vi "Deviation Mode.vi"() -> ()   [LabVIEW 2021]
doc: "Demonstrates how to initialize the bridge, configure measurement parameters, and perform both single and continuous measurements. Additionally this VI demonstrates configuration and execution of deviation mode measurements."
uses:
  <vilib>/Utility/file.llb/Write To Spreadsheet File (string).vi
  Andeen-Hagerling 2700A.lvlib
panel:
  in  "Clear":bool
  in  "Save":bool
  out "measurement buffer":string[](array[string])
  out "cap graph data":dbl[](array[numeric])
  out "loss graph data":dbl[](array[numeric])
  out "time graph data":timestamp[](array[timestamp])
  in  "cancel measure":bool
  in  "cancel dev init":bool
  out "Loss Analog Output":cluster{cluster{dbl, dbl}[]}[](graph)
  out "Capacitance Analog Output":cluster{cluster{dbl, dbl}[]}[](graph)
  out "aout point":T1
  in  "aout bias":T2
  in  "aout span":T3
  in  "aout source":T4 {"aout source cap" items=["DEV", "BIAS", "GROUND"]; "aout source loss" items=["DEV", "BIAS", "GROUND"]}
  in  "aout limit":T5
  in  "aout limit error":T6
  in  "aout cfactor":cluster{"cfactor cap":dbl, "cfactor loss":dbl}
  in  "aout bounds":T7
  out "Interface Information:Interface Type":u16(ring)=1 items=["GPIB"=1, "VXI"=2, "GPIB-VXI"=3, "Serial"=4, "PXI"=5, "TCPIP"=6, "USB"=7, "FireWire"=9]
  out "V 2":string
  out "Hz 2":string
  out "Capacitance Graph":cluster{timestamp[], dbl[]}(graph)
  out "Loss Graph":cluster{timestamp[], dbl[]}(graph)
  in  "Continuous":bool
  in  "dev rollofff":T8
  in  "dev format":T9
  in  "dev average":dbl
  in  "dev point auto":cluster{"cap":bool, "loss":bool}
  in  "dev fetch":bool
  in  "dev position":T10
  in  "dev bounds":T11
  out "deviation region":cluster{cluster{dbl, dbl}[]}[](graph)
  in  "dev margin":dbl
  in  "dev span":cluster{"dev span cap":dbl, "dev span loss":dbl}
  in  "dev point":T12
  out "bridge error":T13
  in  "deviation mode":bool
  out "Bridge Status":string
  out "Error Message":string
  out "V":string
  out "Hz":string
  out "pF":string
  in  "units":i32(ring)=1 items=["NS"=1, "DS"=2, "KO"=3, "GO"=4, "JP"=5]
  out "Applied Voltage":dbl format="%#_10f"
  out "Firmware Revision:":string
  in  "Maximum Applied Voltage":dbl=15.0
  in  "Average\nExponent":i32=4
  in  "Bridge Frequency":dbl=1000.0
  in  "stop":bool
  out "greater than":string
  out "Loss":dbl format="%#_10f"
  out "Measurement Frequency":dbl format="%#_10f"
  out "Capacitance":dbl format="%#_10f"
  out "measurement results":T14 {"Loss" format="%#_10f"; "Capacitance" format="%#_10f"; "Frequency" format="%#_8f"}
  in  "Measure":bool
  # "Deviation Mode Parameters"
  # "AH2700A ULTRA-PRECISION CAPACITANCE BRIDGE"
  # "Measurement Parameters"
  # "Measurement Results"
  # "Analog Out Parameters"
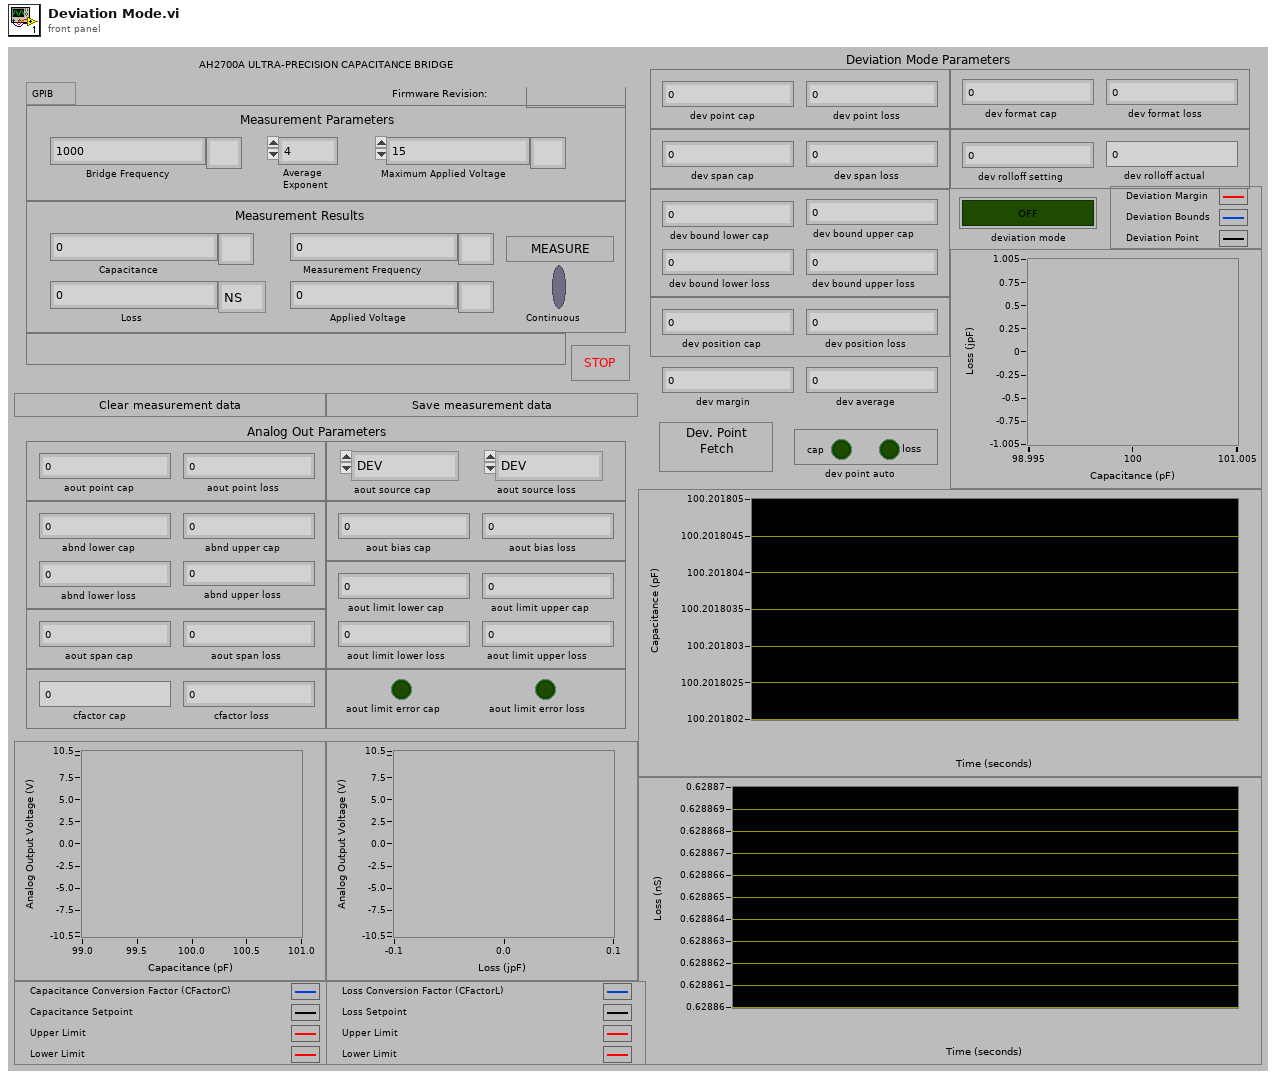
[diagram p1: front panel]
types:
  T1 = cluster{"aout point cap":dbl, "aout point loss":dbl}
  T2 = cluster{"aout bias cap":dbl, "aout bias loss":dbl}
  T3 = cluster{"aout span cap":dbl, "aout span loss":dbl}
  T4 = cluster{"aout source cap":u16, "aout source loss":u16}
  T5 = cluster{"aout limit upper cap":dbl, "aout limit upper loss":dbl, "aout limit lower cap":dbl, "aout limit lower loss":dbl}
  T6 = cluster{"aout limit error cap":bool, "aout limit error loss":bool}
  T7 = cluster{"abnd upper cap":dbl, "abnd upper loss":dbl, "abnd lower cap":dbl, "abnd lower loss":dbl}
  T8 = cluster{"dev rolloff setting":dbl, "dev rolloff actual":dbl}
  T9 = cluster{"dev format cap":i32, "dev format loss":i32}
  T10 = cluster{"dev position cap":dbl, "dev position loss":dbl}
  T11 = cluster{"dev bound upper cap":dbl, "dev bound upper loss":dbl, "dev bound lower cap":dbl, "dev bound lower loss":dbl}
  T12 = cluster{"dev point cap":dbl, "dev point loss":dbl}
  T13 = cluster{"error message":string, "error code":i32}
  T14 = cluster{"Error":i32, "Frequency":dbl, "Capacitance":dbl, "Loss":dbl, "GreaterThan":bool, "Voltage":dbl}
  T15 = cluster{"Baud Rate":u32, "Parity":u16, "Data Bits":u16, "Stop Bits":u16, "Flow Control":u16}
  T16 = cluster{"frequency":dbl, "average":i32, "voltage":dbl, "units":i32, "dev mode":bool, "dev point auto":cluster{"dev point auto cap":bool, "dev point auto loss":bool}, "dev parameters":cluster{"dev bounds":cluster{"dev bound upper cap":dbl, "dev bound upper loss":dbl, "dev bound lower cap":dbl, "dev bound lower loss":dbl}, "dev point":cluster{"dev point cap":dbl, "dev point loss":dbl}, "dev position":cluster{"dev position cap":dbl, "dev position loss":dbl}, "dev span":cluster{"dev span cap":dbl, "dev span loss":dbl}, "dev margin":dbl}, "dev average":dbl, "dev format":cluster{"dev format cap":i32, "dev format loss":i32}, "dev rollofff":cluster{"dev rolloff setting":dbl, "dev rolloff actual":dbl}, "aout bias":cluster{"ABiasC":dbl, "ABiasL":dbl}, "aout bounds":cluster{"ABndUpC":dbl, "ABndUpL":dbl, "ABndLoC":dbl, "ABndLoL":dbl}, "aout cfactor":cluster{"CFactorC":dbl, "CFactorL":dbl}, "aout limit error":cluster{"ALimErrC":bool, "ALimErrL":bool}, "aout limit":cluster{"ALimUpC":dbl, "ALimUpL":dbl, "ALimLoC":dbl, "ALimLoL":dbl}, "aout source":cluster{"ASourceC (0:DEV)":u16, "ASourceL (0:DEV)":u16}, "aout span":cluster{"ASpanC (20.0)":dbl, "ASpanL (20.0)":dbl}, "aout point":cluster{"APointC":dbl, "APointL":dbl}}
  T17 = cluster{"dev point auto cap":bool, "dev point auto loss":bool}
  T18 = cluster{"dev bounds":cluster{"dev bound upper cap":dbl, "dev bound upper loss":dbl, "dev bound lower cap":dbl, "dev bound lower loss":dbl}, "dev point":cluster{"dev point cap":dbl, "dev point loss":dbl}, "dev position":cluster{"dev position cap":dbl, "dev position loss":dbl}, "dev span":cluster{"dev span cap":dbl, "dev span loss":dbl}, "dev margin":dbl}
  T19 = cluster{"ABndUpC":dbl, "ABndUpL":dbl, "ABndLoC":dbl, "ABndLoL":dbl}
  T20 = cluster{"ALimUpC":dbl, "ALimUpL":dbl, "ALimLoC":dbl, "ALimLoL":dbl}
  T21 = cluster{"ASpanC (20.0)":dbl, "ASpanL (20.0)":dbl}
  T22 = cluster{"ASourceC (0:DEV)":u16, "ASourceL (0:DEV)":u16}
  T23 = cluster{"dev point cap":bool, "dev point loss":bool}
  T24 = cluster{"dev span cap":bool, "dev span loss":bool}
  T25 = cluster{"dev bound upper cap":bool, "dev bound upper loss":bool, "dev bound lower cap":bool, "dev bound lower loss":bool}
  T26 = cluster{"dev position cap":bool, "dev position loss":bool}
  T27 = cluster{"dev format cap":bool, "dev format loss":bool}
  T28 = cluster{"dev rolloff setting":bool, "dev rolloff actual":bool}
  T29 = cluster{"aout bias cap":bool, "aout bias loss":bool}
  T30 = cluster{"abnd upper cap":bool, "abnd upper loss":bool, "abnd lower cap":bool, "abnd lower loss":bool}
  T31 = cluster{"aout limit upper cap":bool, "aout limit upper loss":bool, "aout limit lower cap":bool, "aout limit lower loss":bool}
  T32 = cluster{"aout span cap":bool, "aout span loss":bool}
  T33 = cluster{"aout source cap":bool, "aout source loss":bool}
  T34 = cluster{"error":i32, "frequency":dbl, "capacitance":dbl, "loss":dbl, "greater than":bool, "voltage":dbl}
  T35 = cluster{"time graph data":timestamp[], "cap graph data":dbl[]}
  T36 = cluster{"time graph data":timestamp[], "loss graph data":dbl[]}
  T37 = cluster{"aout bounds":cluster{"ABndUpC":dbl, "ABndUpL":dbl, "ABndLoC":dbl, "ABndLoL":dbl}, "aout cfactor":cluster{"CFactorC":dbl, "CFactorL":dbl}, "aout span":cluster{"ASpanC":dbl, "ASpanL":dbl}, "aout point":cluster{"APointC":dbl, "APointL":dbl}}
  T38 = cluster{"error code":i32, "frequency":dbl, "capacitance":dbl, "loss":dbl, "greater than":bool, "voltage":dbl}
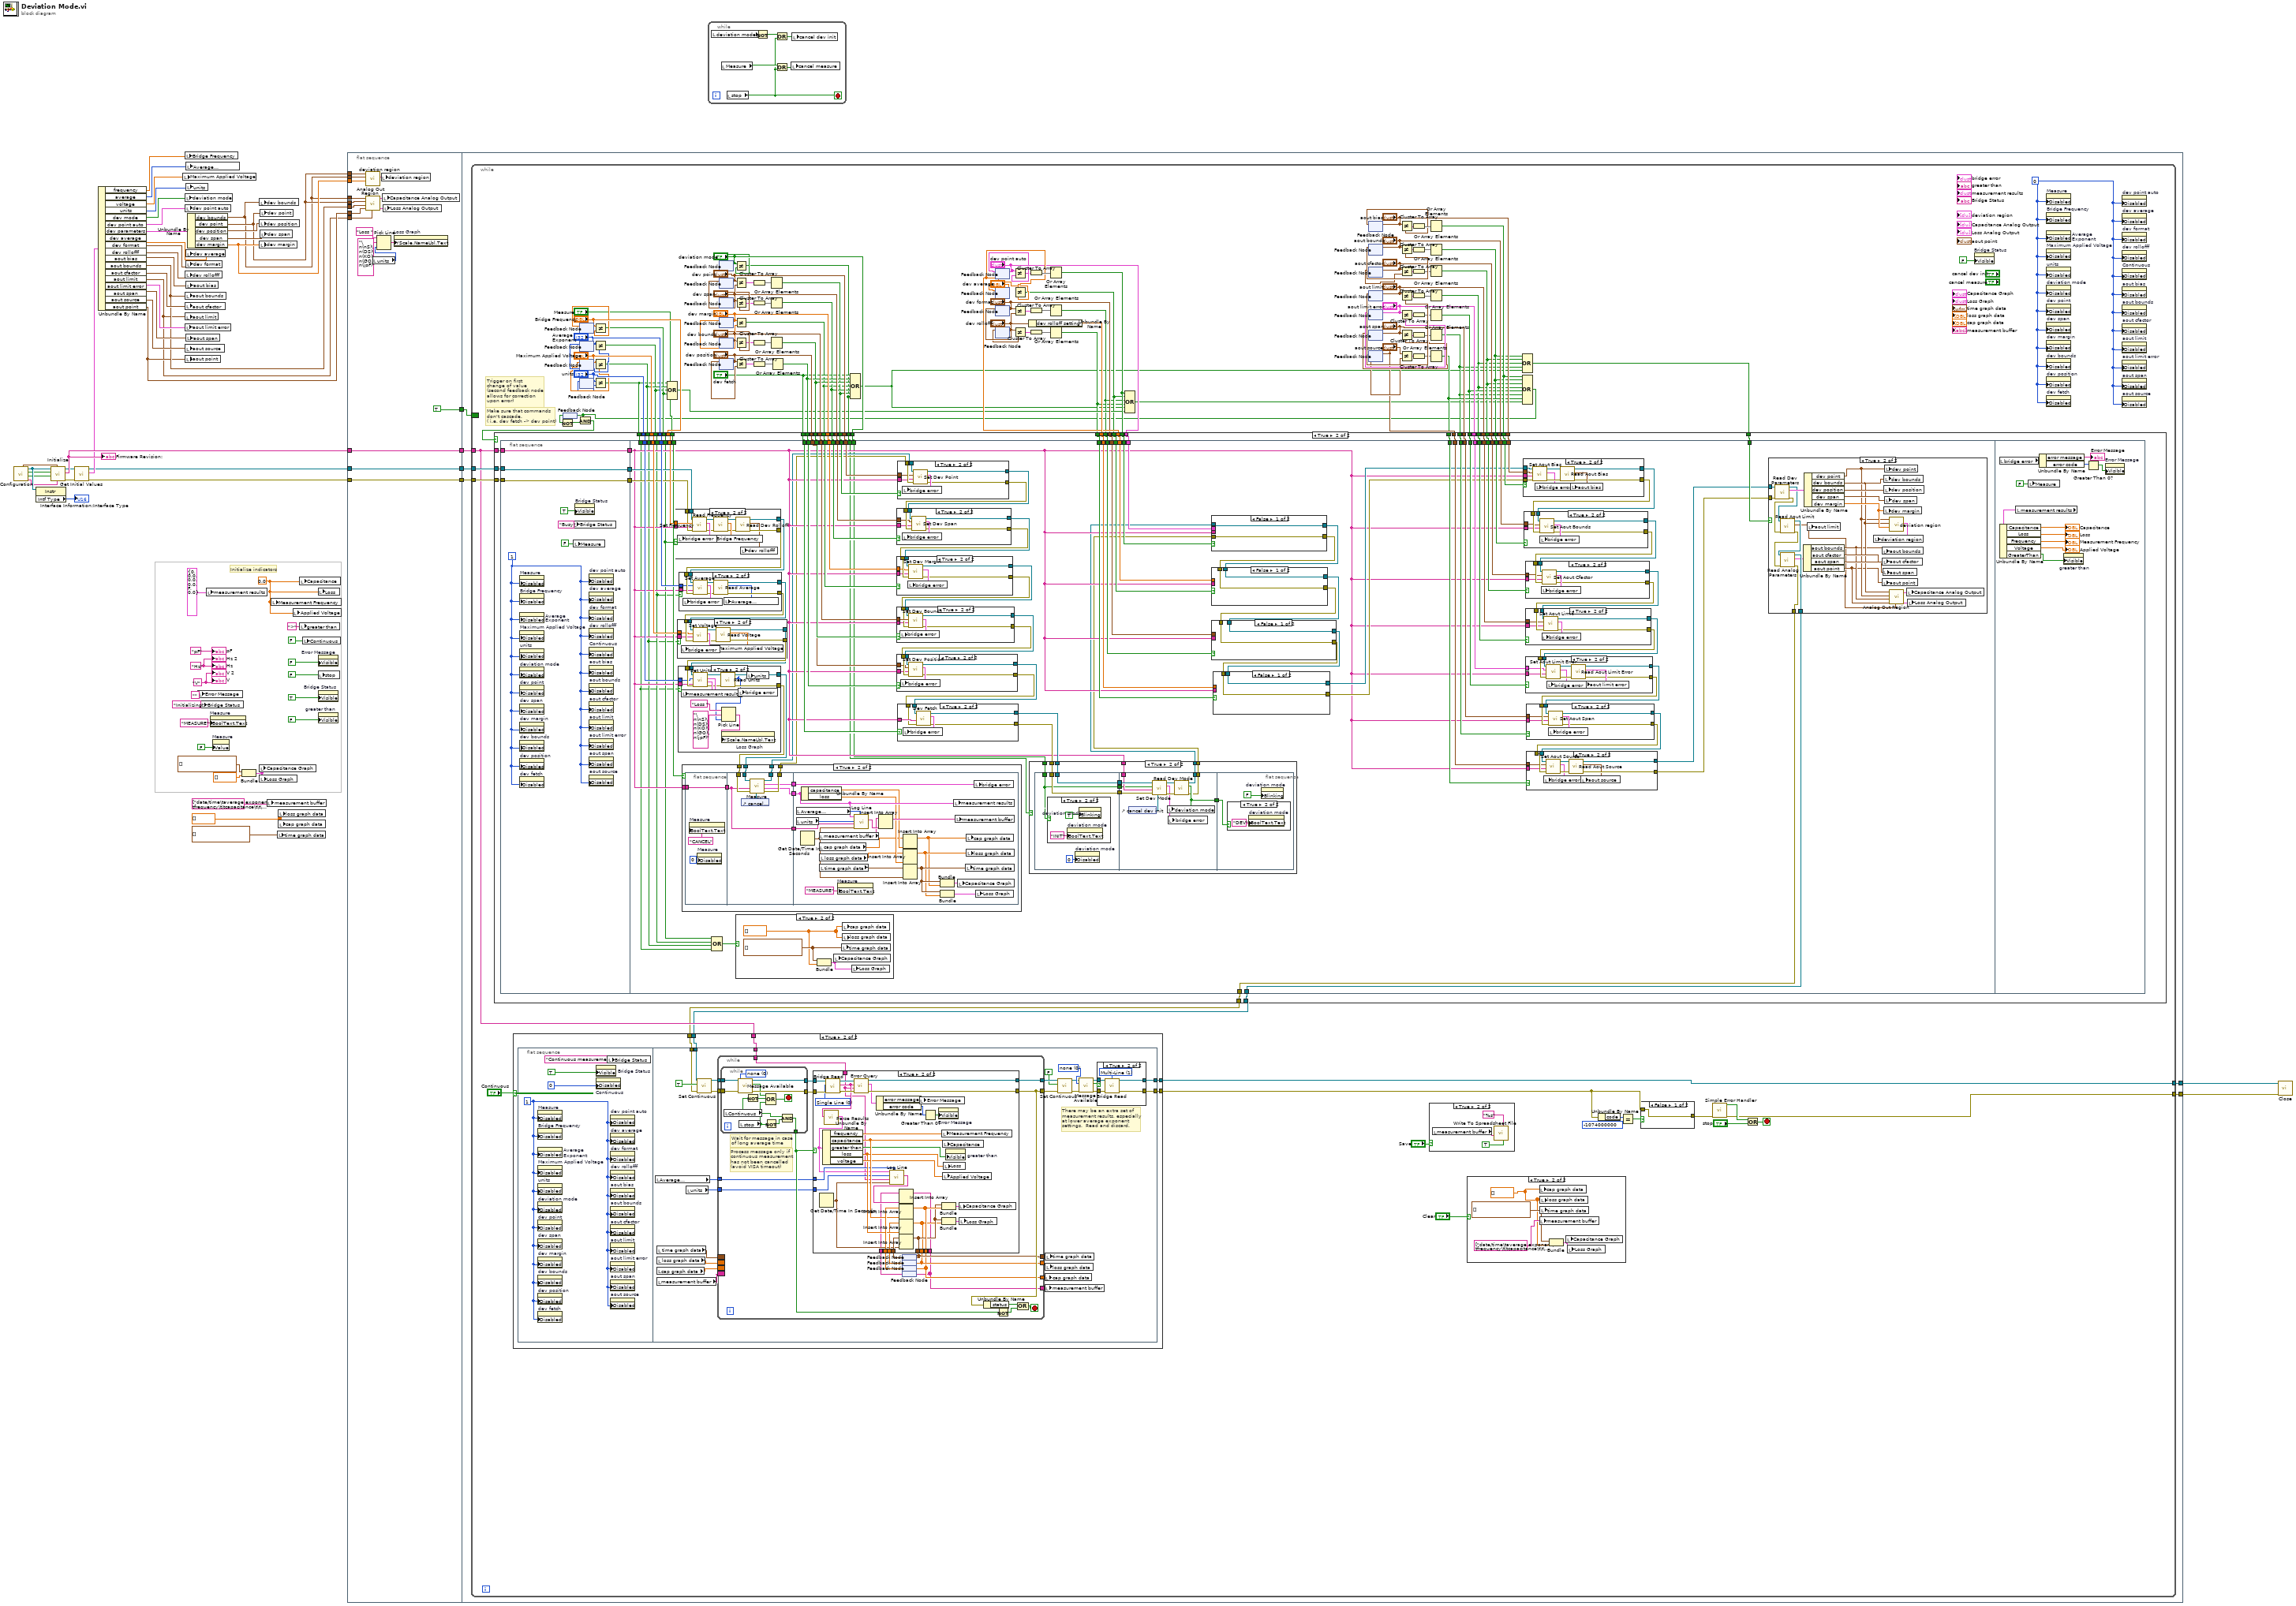
[diagram p0: block diagram]
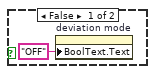
[diagram p11: hidden frame]
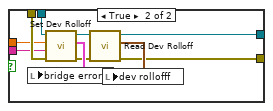
[diagram p20: hidden frame]
diagram:
  w2 = dbl[] []
  w42 = "V" ("V")
  w43 = "Hz" ("Hz")
  w57 = 0.0 ("Capacitance")
  # "Initialize indicators"
  n1 = call "Configuration.vi"() -> ("firmware version"=w9:string, "Reset"=w14:bool, "ID Query"=w10:bool, "VISA resource name out"=w41:refnum<visa-resource-name>, "serial configuration out"=w62:T15)  [unwired: 7 in]
  n2 = property class="Instr"(reference=w41) -> ("Intf Type"=→"Interface Information:Interface Type":u16)  [unwired: 1 in, 2 out]
  n3 = call "Initialize.vi"("firmware revision"=w9, "Serial Configuration"=w62, "Reset (True)"=w14, "ID Query (True)"=w10, "VISA resource name"=w41) -> ("error out"=w38:errorcluster, "firmware revision"=w47:string, "VISA resource name out"=w39:refnum<visa-resource-name>)  [unwired: 4 in]
  "Firmware Revision:" <- w47
  n4 = call "Get Initial Values.vi"("error in (no error)"=w38, "VISA resource name"=w39) -> ("error out"=w27:errorcluster, "initial values"=w37:T16, "VISA resource name out"=w26:refnum<visa-resource-name>)  [unwired: 7 in]
  n5 = Unbundle By Name(w37) -> ("frequency"=w23:dbl, "average"=w36:i32, "voltage"=w35:dbl, "units"=w34:i32, "dev mode"=w33:bool, "dev point auto"=w32:T17, "dev parameters"=w31:T18, "dev average"=w30:dbl, "dev format"=w29:T9, "dev rollofff"=w28:T8, "aout bias"=w25:cluster{"ABiasC":dbl, "ABiasL":dbl}, "aout bounds"=w18:T19, "aout cfactor"=w22:cluster{"CFactorC":dbl, "CFactorL":dbl}, "aout limit"=w16:T20, "aout limit error"=w21:cluster{"ALimErrC":bool, "ALimErrL":bool}, "aout span"=w20:T21, "aout source"=w19:T22, "aout point"=w17:cluster{"APointC":dbl, "APointL":dbl})
  n6 = local write "Maximum Applied Voltage"(w35) -> ()
  n7 = local write "Bridge Frequency"(w23) -> ()
  n8 = local write "deviation mode"(w33) -> ()
  n9 = local write "aout limit error"(w21) -> ()
  n10 = local write "dev point auto"(w32) -> ()
  n11 = local write "dev rollofff"(w28) -> ()
  n12 = local write "aout bounds"(w18) -> ()
  n13 = local write "aout cfactor"(w22) -> ()
  n14 = local write "aout limit"(w16) -> ()
  n15 = local write "aout source"(w19) -> ()
  n16 = local write "aout point"(w17) -> ()
  n17 = local write "Average\nExponent"(w36) -> ()
  n18 = local write "units"(w34) -> ()
  n19 = local write "dev average"(w30) -> ()
  n20 = local write "dev format"(w29) -> ()
  n21 = local write "aout bias"(w25) -> ()
  n22 = local write "aout span"(w20) -> ()
  n23 = Unbundle By Name(w31) -> ("dev bounds"=w6:T11, "dev point"=w7:T12, "dev position"=w49:T10, "dev span"=w48:cluster{"dev span cap":dbl, "dev span loss":dbl}, "dev margin"=w8:dbl)
  n24 = local write "Error Message"("") -> ()
  n25 = local write "Bridge Status"("Initializing" ("Error Message")) -> ()
  n26 = local write "measurement results"(T14 {"Error"=0, "Frequency"=0.0, "Capacitance"=0.0, "Loss"=0.0, "GreaterThan"=FALSE, "Voltage"=0.0} ("measurement results")) -> ()
  n27 = property on="Measure" class="Bool (strict)"("BoolText.Text"="MEASURE" ("Boolean Text.Text")) -> ()  [unwired: 2 in, 2 out]
  n28 = property on="Measure" class="Bool (strict)"("Value"=FALSE ("Measure")) -> ()  [unwired: 2 in, 2 out]
  n29 = Bundle(timestamp[] [], dbl[] []) -> (w44:cluster{timestamp[], dbl[]})  [unwired: 1 in]
  n30 = local write "Capacitance Graph"(w44) -> ()
  n31 = local write "dev bounds"(w6) -> ()
  n32 = local write "dev position"(w49) -> ()
  n33 = local write "dev margin"(w8) -> ()
  n34 = local write "Loss Graph"(w44) -> ()
  n35 = local write "dev point"(w7) -> ()
  n36 = local write "dev span"(w48) -> ()
  n37 = local write "measurement buffer"(string[] ["date/time\taverage exponent\tfrequency\t\tcapacitance\t\t\tloss\t\tvoltage\t\terror code\terror message"]) -> ()
  n38 = local write "Measurement Frequency"(w57) -> ()
  n39 = local write "time graph data"(timestamp[] []) -> ()
  n40 = local write "loss graph data"(w2) -> ()
  n41 = local write "cap graph data"(w2) -> ()
  n42 = local write "Applied Voltage"(w57) -> ()
  n43 = local write "Capacitance"(w57) -> ()
  n44 = local write "greater than"(">" ("greater than")) -> ()
  n45 = local write "Continuous"(FALSE ("Continuous")) -> ()
  n46 = local write "Loss"(w57) -> ()
  n47 = property on="Error Message" class="Str"("Visible"=FALSE) -> ()  [unwired: 2 in, 2 out]
  n48 = local write "stop"(FALSE ("stop")) -> ()
  n49 = property on="Bridge Status" class="Str"("Visible"=TRUE) -> ()  [unwired: 2 in, 2 out]
  n50 = property on="greater than" class="Str"("Visible"=FALSE) -> ()  [unwired: 2 in, 2 out]
  n51 = flat-sequence {
    tunnel: w27 -> [w79]
    tunnel: w26 -> [w80]
    tunnel: w47 -> [w81]
    tunnel: [w81] -> w52
    tunnel: [w80] -> w51
    tunnel: [w79] -> w50
    tunnel: w6 -> [w77]
    tunnel: w7 -> [w76]
    tunnel: w8 -> [w75]
    tunnel: [TRUE] -> w24
    tunnel: w6 -> [w73]
    tunnel: w7 -> [w72]
    tunnel: w18 -> [w71]
    tunnel: w17 -> [w70]
    tunnel: w16 -> [w63]
    tunnel: [w87] -> w60
    tunnel: [w86] -> w59
    tunnel: w52 -> [w85]
    tunnel: w51 -> [w84]
    tunnel: w50 -> [w83]
    tunnel: w24 -> [w82]
    frame #0 {
      n52 = call "deviation region.vi"("dev margin"=w75, "dev bounds"=w77, "dev point"=w76) -> ("deviation region"=w78:cluster{cluster{dbl, dbl}[]}[])  [unwired: 8 in]
      n53 = call "Analog Out Region.vi"("aout limit"=w63, "aout point"=w70, "aout bounds"=w71, "dev point"=w72, "dev bounds"=w73) -> ("Loss Analog Output"=w68:cluster{cluster{dbl, dbl}[]}[], "Capacitance Analog Output"=w69:cluster{cluster{dbl, dbl}[]}[])  [unwired: 5 in]
      n54 = local read "units"() -> (w65:i32)
      n55 = Pick Line(string ("")="Loss ", multi-line string="\n(nS)\n(DS)\n(KO)\n(GO)\n(jpF)", line index=w65) -> (output string=w64:string)
      n56 = local write "deviation region"(w78) -> ()
      n57 = local write "Capacitance Analog Output"(w69) -> ()
      n58 = local write "Loss Analog Output"(w68) -> ()
      n59 = property on="Loss Graph" class="XYGraph (strict)"("YScale.NameLbl.Text"=w64) -> ()  [unwired: 2 in, 2 out]
    }
    frame #1 {
      n60 = while {
        tunnel: w84 -> [w209]
        tunnel: w83 -> [w208]
        tunnel: [w204] -> w87
        tunnel: [w160] -> w86
        tunnel: w85 -> [w159]
        border: w82 -> [_]
        stop <- w205 stop-if-true
        w102 = u8 0 ("Disabled")
        # "Trigger on first\nchange of value\n(second feedback node\nallows for correction\nupon error)"
        # "Make sure that commands\ndon't cascade. \n( i.e. dev fetch -> dev point)"
        n61 = feedback #1() -> (w157:bool)
        n62 = Not(x=w157) -> (.not. x?=w158:bool)
        n63 = feedback-in #2("Bridge Frequency") -> ()
        n64 = feedback #2() -> (w192:dbl)  [unwired: 1 in]
        n65 = feedback-in #3("Average\nExponent") -> ()
        n66 = feedback #3() -> (w191:i32)  [unwired: 1 in]
        n67 = feedback-in #4("Maximum Applied Voltage") -> ()
        n68 = feedback #4() -> (w190:dbl)  [unwired: 1 in]
        n69 = feedback-in #5("units") -> ()
        n70 = feedback #5() -> (w189:i32)  [unwired: 1 in]
        n71 = Not Equal?(x="Bridge Frequency", y=w192) -> (x != y?=w150:bool)
        n72 = Not Equal?(x="Average\nExponent", y=w191) -> (x != y?=w149:bool)
        n73 = Not Equal?(x="Maximum Applied Voltage", y=w190) -> (x != y?=w151:bool)
        n74 = Not Equal?(x="units", y=w189) -> (x != y?=w148:bool)
        n75 = Compound Arithmetic op=OR(w148, w151, w149, w150, "Measure") -> (w100:bool)
        n76 = feedback-in #6("deviation mode") -> ()
        n77 = feedback #6() -> (w193:bool)  [unwired: 1 in]
        n78 = feedback-in #7("dev point") -> ()
        n79 = feedback #7() -> (w188:T12)  [unwired: 1 in]
        n80 = feedback-in #8("dev span") -> ()
        n81 = feedback #8() -> (w186:cluster{"dev span cap":dbl, "dev span loss":dbl})  [unwired: 1 in]
        n82 = feedback-in #9("dev margin") -> ()
        n83 = feedback #9() -> (w184:dbl)  [unwired: 1 in]
        n84 = feedback-in #10("dev bounds") -> ()
        n85 = feedback #10() -> (w179:T11)  [unwired: 1 in]
        n86 = feedback-in #11("dev position") -> ()
        n87 = feedback #11() -> (w176:T10)  [unwired: 1 in]
        n88 = Not Equal?(x="deviation mode", y=w193) -> (x != y?=w101:bool)
        n89 = Not Equal?(x="dev point", y=w188) -> (x != y?=w147:T23)
        n90 = Not Equal?(x="dev span", y=w186) -> (x != y?=w146:T24)
        n91 = Not Equal?(x="dev margin", y=w184) -> (x != y?=w145:bool)
        n92 = Not Equal?(x="dev bounds", y=w179) -> (x != y?=w144:T25)
        n93 = Not Equal?(x="dev position", y=w176) -> (x != y?=w143:T26)
        n94 = Cluster To Array(cluster=w147) -> (array=w187:bool[])
        n95 = Cluster To Array(cluster=w146) -> (array=w185:bool[])
        n96 = Cluster To Array(cluster=w144) -> (array=w180:bool[])
        n97 = Cluster To Array(cluster=w143) -> (array=w177:bool[])
        n98 = Or Array Elements(Boolean array=w187) -> (logical OR=w169:bool)
        n99 = Or Array Elements(Boolean array=w185) -> (logical OR=w170:bool)
        n100 = Or Array Elements(Boolean array=w180) -> (logical OR=w171:bool)
        n101 = Or Array Elements(Boolean array=w177) -> (logical OR=w172:bool)
        n102 = Compound Arithmetic op=OR("dev fetch", w172, w171, w145, w170, w169, w101) -> (w94:bool)
        n103 = feedback-in #12("dev point auto") -> ()
        n104 = feedback #12() -> (w153:cluster{"cap":bool, "loss":bool})  [unwired: 1 in]
        n105 = feedback-in #13("dev average") -> ()
        n106 = feedback #13() -> (w155:dbl)  [unwired: 1 in]
        n107 = feedback-in #14("dev format") -> ()
        n108 = feedback #14() -> (w141:T9)  [unwired: 1 in]
        n109 = feedback-in #15("dev rollofff") -> ()
        n110 = feedback #15() -> (w138:T8)  [unwired: 1 in]
        n111 = Not Equal?(x="dev point auto", y=w153) -> (x != y?=w152:cluster{"cap":bool, "loss":bool})
        n112 = Not Equal?(x="dev average", y=w155) -> (x != y?=w99:bool)
        n113 = Not Equal?(x="dev format", y=w141) -> (x != y?=w140:T27)
        n114 = Not Equal?(x="dev rollofff", y=w138) -> (x != y?=w137:T28)
        n115 = Cluster To Array(cluster=w152) -> (array=w174:bool[])
        n116 = Cluster To Array(cluster=w140) -> (array=w165:bool[])
        n117 = Unbundle By Name("dev rollofff") -> ("dev rolloff setting"=w163:dbl)
        n118 = Cluster To Array(cluster=w137) -> (array=w164:bool[])
        n119 = Or Array Elements(Boolean array=w174) -> (logical OR=w167:bool)
        n120 = Or Array Elements(Boolean array=w165) -> (logical OR=w98:bool)
        n121 = Or Array Elements(Boolean array=w164) -> (logical OR=w97:bool)
        n122 = Compound Arithmetic op=OR(w167, w99, w98, w97, w94, w100) -> (w93:bool)
        n123 = feedback-in #16("aout bias") -> ()
        n124 = feedback #16() -> (w134:T2)  [unwired: 1 in]
        n125 = feedback-in #17("aout bounds") -> ()
        n126 = feedback #17() -> (w130:T7)  [unwired: 1 in]
        n127 = feedback-in #18("aout cfactor") -> ()
        n128 = feedback #18() -> (w125:cluster{"cfactor cap":dbl, "cfactor loss":dbl})  [unwired: 1 in]
        n129 = feedback-in #19("aout limit") -> ()
        n130 = feedback #19() -> (w121:T5)  [unwired: 1 in]
        n131 = feedback-in #20("aout limit error") -> ()
        n132 = feedback #20() -> (w117:T6)  [unwired: 1 in]
        n133 = feedback-in #21("aout span") -> ()
        n134 = feedback #21() -> (w113:T3)  [unwired: 1 in]
        n135 = feedback-in #22("aout source") -> ()
        n136 = feedback #22() -> (w109:T4)  [unwired: 1 in]
        n137 = Not Equal?(x="aout bias", y=w134) -> (x != y?=w135:T29)
        n138 = Not Equal?(x="aout bounds", y=w130) -> (x != y?=w131:T30)
        n139 = Not Equal?(x="aout cfactor", y=w125) -> (x != y?=w126:cluster{"cfactor cap":bool, "cfactor loss":bool})
        n140 = Not Equal?(x="aout limit", y=w121) -> (x != y?=w122:T31)
        n141 = Not Equal?(x="aout limit error", y=w117) -> (x != y?=w118:T6)
        n142 = Not Equal?(x="aout span", y=w113) -> (x != y?=w114:T32)
        n143 = Not Equal?(x="aout source", y=w109) -> (x != y?=w110:T33)
        n144 = Cluster To Array(cluster=w135) -> (array=w136:bool[])
        n145 = Cluster To Array(cluster=w131) -> (array=w132:bool[])
        n146 = Cluster To Array(cluster=w126) -> (array=w127:bool[])
        n147 = Cluster To Array(cluster=w122) -> (array=w123:bool[])
        n148 = Cluster To Array(cluster=w118) -> (array=w119:bool[])
        n149 = Cluster To Array(cluster=w114) -> (array=w115:bool[])
        n150 = Cluster To Array(cluster=w110) -> (array=w111:bool[])
        n151 = Or Array Elements(Boolean array=w136) -> (logical OR=w128:bool)
        n152 = Or Array Elements(Boolean array=w132) -> (logical OR=w106:bool)
        n153 = Or Array Elements(Boolean array=w127) -> (logical OR=w105:bool)
        n154 = Or Array Elements(Boolean array=w123) -> (logical OR=w96:bool)
        n155 = Or Array Elements(Boolean array=w119) -> (logical OR=w104:bool)
        n156 = Or Array Elements(Boolean array=w115) -> (logical OR=w95:bool)
        n157 = Or Array Elements(Boolean array=w111) -> (logical OR=w107:bool)
        n158 = case shown="True" "Save" {
          frame False {
          }
          frame True {
            n159 = local read "measurement buffer"() -> (w214:string[])
            n160 = call-poly <vilib>:"Write To Spreadsheet File.vi"("transpose? (no:F)"=TRUE, "format (%s)"="%s", "1D data"=w214) -> ()  [unwired: 5 in, 1 out]
          }
        }
        n161 = case shown="True" "Clear" {
          frame False {
          }
          frame True {
            w210 = dbl[] []
            w213 = timestamp[] [] ("time graph data")
            n162 = local write "cap graph data"(w210) -> ()
            n163 = local write "measurement buffer"(string[] ["date/time\taverage exponent\tfrequency\t\tcapacitance\t\t\tloss\t\tvoltage\t\terror code\terror message"]) -> ()
            n164 = local write "loss graph data"(w210) -> ()
            n165 = local write "time graph data"(w213) -> ()
            n166 = Bundle("time graph data"=w213, w210) -> (w212:cluster{"time graph data":timestamp[], dbl[]})  [unwired: 1 in]
            n167 = local write "Capacitance Graph"(w212) -> ()
            n168 = local write "Loss Graph"(w212) -> ()
          }
        }
        n169 = Compound Arithmetic op=OR(w106, w105, w96, w95, w94) -> (w103:bool)
        n170 = Compound Arithmetic op=OR(w128, w106, w105, w96, w104, w95, w107, w93) -> (w92:bool)
        n171 = feedback-in #1(w92) -> ()
        n172 = And(x=w92, y=w158) -> (x .and. y?=w166:bool)
        n173 = case shown="True" w166 {
          tunnel: w209 -> [w334 w386]
          tunnel: w208 -> [w335 w385]
          tunnel: "Measure" -> [_ w384]
          tunnel: w150 -> [_ w383]
          tunnel: "Bridge Frequency" -> [_ w382]
          tunnel: "Average\nExponent" -> [_ w381]
          tunnel: w149 -> [_ w380]
          tunnel: "Maximum Applied Voltage" -> [_ w379]
          tunnel: w151 -> [_ w378]
          tunnel: "units" -> [_ w377]
          tunnel: w148 -> [_ w376]
          tunnel: w159 -> [_ w374]
          tunnel: w101 -> [_ w373]
          tunnel: "deviation mode" -> [_ w372]
          tunnel: "dev point" -> [_ w371]
          tunnel: w169 -> [_ w370]
          tunnel: "dev span" -> [_ w369]
          tunnel: w170 -> [_ w368]
          tunnel: "dev margin" -> [_ w367]
          tunnel: w145 -> [_ w366]
          tunnel: "dev bounds" -> [_ w365]
          tunnel: w171 -> [_ w364]
          tunnel: "dev position" -> [_ w363]
          tunnel: w172 -> [_ w362]
          tunnel: "dev point auto" -> [_ w361]
          tunnel: w167 -> [_ w360]
          tunnel: "dev fetch" -> [_ w359]
          tunnel: "dev average" -> [_ w358]
          tunnel: w99 -> [_ w357]
          tunnel: "dev format" -> [_ w356]
          tunnel: w98 -> [_ w355]
          tunnel: w163 -> [_ w354]
          tunnel: w97 -> [_ w353]
          tunnel: [w334 w352] -> w89
          tunnel: [w335 w351] -> w88
          tunnel: "aout bias" -> [_ w350]
          tunnel: w128 -> [_ w349]
          tunnel: "aout bounds" -> [_ w348]
          tunnel: w106 -> [_ w347]
          tunnel: "aout cfactor" -> [_ w346]
          tunnel: w105 -> [_ w345]
          tunnel: "aout limit" -> [_ w344]
          tunnel: w96 -> [_ w343]
          tunnel: "aout limit error" -> [_ w342]
          tunnel: w104 -> [_ w341]
          tunnel: "aout span" -> [_ w340]
          tunnel: w95 -> [_ w339]
          tunnel: "aout source" -> [_ w338]
          tunnel: w107 -> [_ w337]
          tunnel: w103 -> [_ w336]
          frame False {
          }
          frame True {
            n174 = flat-sequence {
              tunnel: w385 -> [w394]
              tunnel: w386 -> [w395]
              tunnel: [w395] -> w388
              tunnel: [w394] -> w387
              tunnel: [w392] -> w375
              tunnel: w374 -> [w392]
              tunnel: w384 -> [w410]
              tunnel: w388 -> [w414]
              tunnel: w387 -> [w413]
              tunnel: w383 -> [w399]
              tunnel: w382 -> [w492]
              tunnel: w381 -> [w491]
              tunnel: w380 -> [w398]
              tunnel: w379 -> [w488]
              tunnel: w378 -> [w397]
              tunnel: w377 -> [w484]
              tunnel: w376 -> [w396]
              tunnel: w375 -> [w407]
              tunnel: w373 -> [w403]
              tunnel: w372 -> [w404]
              tunnel: w371 -> [w482]
              tunnel: w370 -> [w481]
              tunnel: w369 -> [w478]
              tunnel: w368 -> [w477]
              tunnel: w367 -> [w474]
              tunnel: w366 -> [w473]
              tunnel: w365 -> [w472]
              tunnel: w364 -> [w469]
              tunnel: w363 -> [w468]
              tunnel: w362 -> [w467]
              tunnel: w361 -> [w464]
              tunnel: w360 -> [w463]
              tunnel: w359 -> [w460]
              tunnel: w358 -> [w459]
              tunnel: w357 -> [w456]
              tunnel: w356 -> [w453]
              tunnel: w355 -> [w452]
              tunnel: w354 -> [w451]
              tunnel: w353 -> [w450]
              tunnel: [w415] -> w352
              tunnel: [w416] -> w351
              tunnel: w350 -> [w447]
              tunnel: w349 -> [w446]
              tunnel: w348 -> [w443]
              tunnel: w347 -> [w442]
              tunnel: w346 -> [w439]
              tunnel: w345 -> [w438]
              tunnel: w344 -> [w435]
              tunnel: w343 -> [w434]
              tunnel: w342 -> [w431]
              tunnel: w341 -> [w430]
              tunnel: w340 -> [w427]
              tunnel: w339 -> [w426]
              tunnel: w338 -> [w423]
              tunnel: w337 -> [w422]
              tunnel: w336 -> [w419]
              frame #0 {
                w390 = u8 1 ("Disabled")
                n175 = property on="Measure" class="Bool (strict)"("Disabled"=w390) -> ()  [unwired: 2 in, 2 out]
                n176 = property on="Bridge Frequency" class="DigNum (strict)"("Disabled"=w390) -> ()  [unwired: 2 in, 2 out]
                n177 = property on="Average\nExponent" class="DigNum (strict)"("Disabled"=w390) -> ()  [unwired: 2 in, 2 out]
                n178 = property on="Maximum Applied Voltage" class="DigNum (strict)"("Disabled"=w390) -> ()  [unwired: 2 in, 2 out]
                n179 = property on="units" class="Ring (strict)"("Disabled"=w390) -> ()  [unwired: 2 in, 2 out]
                n180 = property on="deviation mode" class="Bool (strict)"("Disabled"=w390) -> ()  [unwired: 2 in, 2 out]
                n181 = property on="dev point" class="Clust (strict)"("Disabled"=w390) -> ()  [unwired: 2 in, 2 out]
                n182 = property on="dev span" class="Clust (strict)"("Disabled"=w390) -> ()  [unwired: 2 in, 2 out]
                n183 = property on="dev margin" class="DigNum (strict)"("Disabled"=w390) -> ()  [unwired: 2 in, 2 out]
                n184 = property on="dev bounds" class="Clust (strict)"("Disabled"=w390) -> ()  [unwired: 2 in, 2 out]
                n185 = property on="dev position" class="Clust (strict)"("Disabled"=w390) -> ()  [unwired: 2 in, 2 out]
                n186 = property on="dev fetch" class="Bool"("Disabled"=w390) -> ()  [unwired: 2 in, 2 out]
                n187 = local write "Bridge Status"("Busy" ("Bridge Status")) -> ()
                n188 = local write "Measure"(FALSE ("Measure")) -> ()
                n189 = property on="Bridge Status" class="Str"("Visible"=TRUE) -> ()  [unwired: 2 in, 2 out]
                n190 = property on="dev point auto" class="Clust (strict)"("Disabled"=w390) -> ()  [unwired: 2 in, 2 out]
                n191 = property on="dev average" class="DigNum (strict)"("Disabled"=w390) -> ()  [unwired: 2 in, 2 out]
                n192 = property on="dev format" class="Clust (strict)"("Disabled"=w390) -> ()  [unwired: 2 in, 2 out]
                n193 = property on="dev rollofff" class="Clust (strict)"("Disabled"=w390) -> ()  [unwired: 2 in, 2 out]
                n194 = property on="Continuous" class="Bool (strict)"("Disabled"=w390) -> ()  [unwired: 2 in, 2 out]
                n195 = property on="aout bias" class="Clust (strict)"("Disabled"=w390) -> ()  [unwired: 2 in, 2 out]
                n196 = property on="aout bounds" class="Clust (strict)"("Disabled"=w390) -> ()  [unwired: 2 in, 2 out]
                n197 = property on="aout cfactor" class="Clust (strict)"("Disabled"=w390) -> ()  [unwired: 2 in, 2 out]
                n198 = property on="aout limit" class="Clust (strict)"("Disabled"=w390) -> ()  [unwired: 2 in, 2 out]
                n199 = property on="aout limit error" class="Clust (strict)"("Disabled"=w390) -> ()  [unwired: 2 in, 2 out]
                n200 = property on="aout span" class="Clust (strict)"("Disabled"=w390) -> ()  [unwired: 2 in, 2 out]
                n201 = property on="aout source" class="Clust (strict)"("Disabled"=w390) -> ()  [unwired: 2 in, 2 out]
              }
              frame #1 {
                n202 = case shown="True" w399 {
                  tunnel: w492 -> [_ w781]
                  tunnel: w414 -> [w768 w780]
                  tunnel: w413 -> [w767 w779]
                  tunnel: w407 -> [_ w778]
                  tunnel: [w768 w771] -> w490
                  tunnel: [w767 w770] -> w489
                  frame False {
                  }
                  frame True {
                    n203 = call "Set Frequency.vi"("error in (no error)"=w779, "firmware revision"=w778, "frequency (1000)"=w781, "VISA resource name"=w780) -> ("error out"=w775:errorcluster, "bridge error"=w777:T13, "VISA resource name out"=w776:refnum<visa-resource-name>)  [unwired: 5 in]
                    n204 = local write "bridge error"(w777) -> ()
                    n205 = call "Read Frequency.vi"("error in (no error)"=w775, "VISA resource name"=w776) -> ("error out"=w772:errorcluster, "frequency"=w774:dbl, "VISA resource name out"=w773:refnum<visa-resource-name>)  [unwired: 7 in]
                    n206 = local write "Bridge Frequency"(w774) -> ()
                    n207 = call "Read Dev Rolloff.vi"("error in (no error)"=w772, "VISA resource name"=w773) -> ("error out"=w770:errorcluster, "dev rollofff"=w769:T8, "VISA resource name out"=w771:refnum<visa-resource-name>)  [unwired: 7 in]
                    n208 = local write "dev rollofff"(w769) -> ()
                  }
                }
                n209 = case shown="True" w398 {
                  tunnel: w490 -> [w756 w766]
                  tunnel: w489 -> [w755 w765]
                  tunnel: [w756 w758] -> w486
                  tunnel: [w755 w760] -> w487
                  tunnel: w491 -> [_ w764]
                  tunnel: w407 -> [_ w763]
                  frame False {
                  }
                  frame True {
                    n210 = call "Set Average.vi"("error in (no error)"=w765, "firmware revision"=w763, "average (4)"=w764, "VISA resource name"=w766) -> ("error out"=w761:errorcluster, "bridge error"=w762:T13, "VISA resource name out"=w759:refnum<visa-resource-name>)  [unwired: 5 in]
                    n211 = local write "bridge error"(w762) -> ()
                    n212 = call "Read Average.vi"("error in (no error)"=w761, "VISA resource name"=w759) -> ("error out"=w760:errorcluster, "average"=w757:i32, "VISA resource name out"=w758:refnum<visa-resource-name>)  [unwired: 7 in]
                    n213 = local write "Average\nExponent"(w757) -> ()
                  }
                }
                n214 = case shown="True" w397 {
                  tunnel: w486 -> [w744 w754]
                  tunnel: w487 -> [w743 w753]
                  tunnel: [w744 w748] -> w483
                  tunnel: [w743 w746] -> w485
                  tunnel: w407 -> [_ w752]
                  tunnel: w488 -> [_ w751]
                  frame False {
                  }
                  frame True {
                    n215 = call "Set Voltage.vi"("error in (no error)"=w753, "firmware revision"=w752, "voltage (15)"=w751, "VISA resource name"=w754) -> ("error out"=w747:errorcluster, "bridge error"=w750:T13, "VISA resource name out"=w749:refnum<visa-resource-name>)  [unwired: 5 in]
                    n216 = local write "bridge error"(w750) -> ()
                    n217 = call "Read Voltage.vi"("error in (no error)"=w747, "VISA resource name"=w749) -> ("error out"=w746:errorcluster, "voltage"=w745:dbl, "VISA resource name out"=w748:refnum<visa-resource-name>)  [unwired: 7 in]
                    n218 = local write "Maximum Applied Voltage"(w745) -> ()
                  }
                }
                n219 = case shown="True" w396 {
                  tunnel: w483 -> [w728 w742]
                  tunnel: w485 -> [w727 w741]
                  tunnel: [w728 w733] -> w411
                  tunnel: [w727 w735] -> w412
                  tunnel: w407 -> [_ w740]
                  tunnel: w484 -> [_ w739]
                  frame False {
                  }
                  frame True {
                    n220 = call "Set Units.vi"("error in (no error)"=w741, "firmware revision"=w740, "units (NS)"=w739, "VISA resource name"=w742) -> ("error out"=w736:errorcluster, "measurement results"=w738:T14, "bridge error"=w737:T13, "VISA resource name out"=w734:refnum<visa-resource-name>)  [unwired: 4 in]
                    n221 = local write "measurement results"(w738) -> ()
                    n222 = call "Read Units.vi"("error in (no error)"=w736, "VISA resource name"=w734) -> ("error out"=w735:errorcluster, "units"=w730:i32, "VISA resource name out"=w733:refnum<visa-resource-name>)  [unwired: 7 in]
                    n223 = Pick Line(string ("")="Loss ", multi-line string="\n(nS)\n(DS)\n(KO)\n(GO)\n(jpF)", line index=w730) -> (output string=w729:string)
                    n224 = property on="Loss Graph" class="XYGraph (strict)"("YScale.NameLbl.Text"=w729) -> ()  [unwired: 2 in, 2 out]
                    n225 = local write "bridge error"(w737) -> ()
                    n226 = local write "units"(w730) -> ()
                  }
                }
                n227 = case shown="True" w410 {
                  tunnel: w407 -> [_ w792]
                  tunnel: w412 -> [w783 w790]
                  tunnel: w411 -> [w782 w789]
                  tunnel: [w782 w788] -> w405
                  tunnel: [w783 w787] -> w406
                  frame False {
                  }
                  frame True {
                    n228 = flat-sequence {
                      tunnel: w792 -> [w793]
                      tunnel: [w793] -> w791
                      tunnel: w791 -> [w796]
                      tunnel: w790 -> [w803]
                      tunnel: w789 -> [w802]
                      tunnel: [w801] -> w788
                      tunnel: [w800] -> w787
                      tunnel: [w798] -> w786
                      tunnel: [w797] -> w785
                      tunnel: [w796] -> w784
                      tunnel: w786 -> [w819]
                      tunnel: w785 -> [w822]
                      tunnel: w784 -> [w818]
                      frame #0 {
                        n229 = property on="Measure" class="Bool (strict)"("BoolText.Text"="CANCEL" ("Label.Text")) -> ()  [unwired: 2 in, 2 out]
                        n230 = property on="Measure" class="Bool (strict)"("Disabled"=u8 0) -> ()  [unwired: 2 in, 2 out]
                      }
                      frame #1 {
                        n231 = control-ref of="cancel measure"() -> (w799:refnum<vi>)
                        n232 = call "Measure.vi"("cancel refnum"=w799, "error in (no error)"=w803, "firmware revision"=w796, "VISA resource name"=w802) -> ("error out"=w800:errorcluster, "measurement results"=w798:T34, "bridge error"=w797:T13, "VISA resource name out"=w801:refnum<visa-resource-name>)  [unwired: 3 in]
                      }
                      frame #2 {
                        n233 = local read "Average\nExponent"() -> (w821:i32)
                        n234 = local read "units"() -> (w820:i32)
                        n235 = Get Date/Time In Seconds() -> (seconds since 1Jan1904=w812:timestamp)
                        n236 = Unbundle By Name(w819) -> ("capacitance"=w814:dbl, "loss"=w813:dbl)
                        n237 = local read "measurement buffer"() -> (w816:string[])
                        n238 = local read "cap graph data"() -> (w811:dbl[])
                        n239 = local read "loss graph data"() -> (w810:dbl[])
                        n240 = local read "time graph data"() -> (w809:timestamp[])
                        n241 = property on="Measure" class="Bool (strict)"("BoolText.Text"="MEASURE" ("Label.Text")) -> ()  [unwired: 2 in, 2 out]
                        n242 = call "Log Line.vi"("average exponent"=w821, "current time"=w812, "firmware revision"=w818, "units"=w820, "measurement results"=w819) -> ("log line"=w817:string)  [unwired: 6 in]
                        n243 = Insert Into Array(array=w816, new element=w817) -> (w815:string[])  [unwired: 1 in]
                        n244 = Insert Into Array(array=w811, new element=w814) -> (w806:dbl[])  [unwired: 1 in]
                        n245 = Insert Into Array(array=w810, new element=w813) -> (w807:dbl[])  [unwired: 1 in]
                        n246 = Insert Into Array(array=w809, new element=w812) -> (w808:timestamp[])  [unwired: 1 in]
                        n247 = Bundle("time graph data"=w808, "cap graph data"=w806) -> (w805:T35)  [unwired: 1 in]
                        n248 = Bundle("time graph data"=w808, "loss graph data"=w807) -> (w804:T36)  [unwired: 1 in]
                        n249 = local write "measurement results"(w819) -> ()
                        n250 = local write "measurement buffer"(w815) -> ()
                        n251 = local write "Capacitance Graph"(w805) -> ()
                        n252 = local write "time graph data"(w808) -> ()
                        n253 = local write "cap graph data"(w806) -> ()
                        n254 = local write "loss graph data"(w807) -> ()
                        n255 = local write "bridge error"(w822) -> ()
                        n256 = local write "Loss Graph"(w804) -> ()
                      }
                    }
                  }
                }
                n257 = Compound Arithmetic op=OR(w399, w398, w397, w396) -> (w400:bool)
                n258 = case shown="True" w400 {
                  frame False {
                  }
                  frame True {
                    w493 = dbl[] []
                    w494 = timestamp[] [] ("time graph data")
                    n259 = Bundle("time graph data"=w494, w493) -> (w495:cluster{"time graph data":timestamp[], dbl[]})  [unwired: 1 in]
                    n260 = local write "Capacitance Graph"(w495) -> ()
                    n261 = local write "time graph data"(w494) -> ()
                    n262 = local write "cap graph data"(w493) -> ()
                    n263 = local write "loss graph data"(w493) -> ()
                    n264 = local write "Loss Graph"(w495) -> ()
                  }
                }
                n265 = case shown="True" w481 {
                  tunnel: w405 -> [w718 w725]
                  tunnel: w406 -> [w719 w724]
                  tunnel: [w718 w721] -> w480
                  tunnel: [w719 w720] -> w479
                  tunnel: w482 -> [_ w723]
                  tunnel: w407 -> [_ w722]
                  frame False {
                  }
                  frame True {
                    n266 = call "Set Dev Point.vi"("error in (no error)"=w724, "firmware revision"=w722, "dev point"=w723, "VISA resource name"=w725) -> ("error out"=w720:errorcluster, "bridge error"=w726:T13, "VISA resource name out"=w721:refnum<visa-resource-name>)  [unwired: 5 in]
                    n267 = local write "bridge error"(w726) -> ()
                  }
                }
                n268 = case shown="True" w477 {
                  tunnel: w480 -> [w710 w716]
                  tunnel: w479 -> [w709 w715]
                  tunnel: [w710 w711] -> w476
                  tunnel: [w709 w712] -> w475
                  tunnel: w407 -> [_ w714]
                  tunnel: w478 -> [_ w713]
                  frame False {
                  }
                  frame True {
                    n269 = call "Set Dev Span.vi"("error in (no error)"=w715, "firmware revision"=w714, "dev span"=w713, "VISA resource name"=w716) -> ("error out"=w712:errorcluster, "bridge error"=w717:T13, "VISA resource name out"=w711:refnum<visa-resource-name>)  [unwired: 5 in]
                    n270 = local write "bridge error"(w717) -> ()
                  }
                }
                n271 = case shown="True" w473 {
                  tunnel: w476 -> [w701 w707]
                  tunnel: [w701 w702] -> w470
                  tunnel: [w700 w703] -> w471
                  tunnel: w475 -> [w700 w706]
                  tunnel: w407 -> [_ w705]
                  tunnel: w474 -> [_ w704]
                  frame False {
                  }
                  frame True {
                    n272 = call "Set Dev Margin.vi"("error in (no error)"=w706, "firmware revision"=w705, "dev margin (1.0)"=w704, "VISA resource name"=w707) -> ("error out"=w703:errorcluster, "bridge error"=w708:T13, "VISA resource name out"=w702:refnum<visa-resource-name>)  [unwired: 5 in]
                    n273 = local write "bridge error"(w708) -> ()
                  }
                }
                n274 = case shown="True" w469 {
                  tunnel: w472 -> [_ w699]
                  tunnel: w470 -> [w692 w698]
                  tunnel: w471 -> [w691 w697]
                  tunnel: w407 -> [_ w696]
                  tunnel: [w691 w694] -> w466
                  tunnel: [w692 w693] -> w465
                  frame False {
                  }
                  frame True {
                    n275 = call "Set Dev Bounds.vi"("error in (no error)"=w697, "firmware revision"=w696, "dev bounds"=w699, "VISA resource name"=w698) -> ("error out"=w694:errorcluster, "bridge error"=w695:T13, "VISA resource name out"=w693:refnum<visa-resource-name>)  [unwired: 4 in]
                    n276 = local write "bridge error"(w695) -> ()
                  }
                }
                n277 = case shown="True" w467 {
                  tunnel: w465 -> [w683 w690]
                  tunnel: w466 -> [w682 w689]
                  tunnel: w407 -> [_ w687]
                  tunnel: w468 -> [_ w686]
                  tunnel: [w682 w684] -> w461
                  tunnel: [w683 w685] -> w462
                  frame False {
                  }
                  frame True {
                    n278 = call "Set Dev Position.vi"("error in (no error)"=w689, "firmware revision"=w687, "dev position"=w686, "VISA resource name"=w690) -> ("error out"=w684:errorcluster, "bridge error"=w688:T13, "VISA resource name out"=w685:refnum<visa-resource-name>)  [unwired: 5 in]
                    n279 = local write "bridge error"(w688) -> ()
                  }
                }
                n280 = case shown="True" w460 {
                  tunnel: w407 -> [_ w681]
                  tunnel: [w675 w677] -> w408
                  tunnel: [w674 w676] -> w409
                  tunnel: w462 -> [w675 w679]
                  tunnel: w461 -> [w674 w678]
                  frame False {
                  }
                  frame True {
                    n281 = call "Dev Fetch.vi"("error in (no error)"=w678, "firmware revision"=w681, "VISA resource name"=w679) -> ("error out"=w676:errorcluster, "bridge error"=w680:T13, "VISA resource name out"=w677:refnum<visa-resource-name>)  [unwired: 6 in]
                    n282 = local write "bridge error"(w680) -> ()
                  }
                }
                n283 = case shown="True" w403 {
                  tunnel: w409 -> [w496 w507]
                  tunnel: w408 -> [w497 w505]
                  tunnel: w407 -> [_ w503]
                  tunnel: w404 -> [_ w502]
                  tunnel: [w497 w499] -> w402
                  tunnel: [w496 w498] -> w401
                  frame False {
                  }
                  frame True {
                    n284 = flat-sequence {
                      tunnel: w507 -> [w510]
                      tunnel: [w510] -> w506
                      tunnel: w505 -> [w511]
                      tunnel: [w511] -> w504
                      tunnel: w502 -> [w509]
                      tunnel: [w509] -> w500
                      tunnel: w506 -> [w521]
                      tunnel: w504 -> [w520]
                      tunnel: w503 -> [w519]
                      tunnel: [w518] -> w501
                      tunnel: w500 -> [w517]
                      tunnel: [w515] -> w499
                      tunnel: [w514] -> w498
                      tunnel: w501 -> [w525]
                      frame #0 {
                        n285 = case shown="True" w509 {
                          frame False {
                          }
                          frame True {
                            n286 = property on="deviation mode" class="Bool (strict)"("BoolText.Text"="INIT" ("Boolean Text.Text")) -> ()  [unwired: 2 in, 2 out]
                            n287 = property on="deviation mode" class="Bool (strict)"("Blinking"=TRUE) -> ()  [unwired: 2 in, 2 out]
                          }
                        }
                        n288 = property on="deviation mode" class="Bool (strict)"("Disabled"=u8 0) -> ()  [unwired: 2 in, 2 out]
                      }
                      frame #1 {
                        n289 = control-ref of="cancel dev init"() -> (w516:refnum<vi>)
                        n290 = call "Set Dev Mode.vi"("cancel refnum"=w516, "error in (no error)"=w521, "firmware revision"=w519, "dev mode"=w517, "VISA resource name"=w520) -> ("error out"=w524:errorcluster, "bridge error"=w522:T13, "VISA resource name out"=w523:refnum<visa-resource-name>)  [unwired: 4 in]
                        n291 = local write "bridge error"(w522) -> ()
                        n292 = call "Read Dev Mode.vi"("error in (no error)"=w524, "VISA resource name"=w523) -> ("error out"=w514:errorcluster, "dev mode"=w518:bool, "VISA resource name out"=w515:refnum<visa-resource-name>)  [unwired: 7 in]
                        n293 = local write "deviation mode"(w518) -> ()
                      }
                      frame #2 {
                        n294 = case shown="True" w525 {
                          frame False {
                            n295 = property on="deviation mode" class="Bool (strict)"("BoolText.Text"="OFF" ("Boolean Text.Text")) -> ()  [unwired: 2 in, 2 out]
                          }
                          frame True {
                            n296 = property on="deviation mode" class="Bool (strict)"("BoolText.Text"="DEV" ("Boolean Text.Text")) -> ()  [unwired: 2 in, 2 out]
                          }
                        }
                        n297 = property on="deviation mode" class="Bool (strict)"("Blinking"=FALSE) -> ()  [unwired: 2 in, 2 out]
                      }
                    }
                  }
                }
                n298 = case shown="False" w463 {
                  tunnel: w407 -> [_ w673]
                  tunnel: w464 -> [_ w669]
                  tunnel: [w662 w667] -> w458
                  tunnel: [w663 w666] -> w457
                  tunnel: w402 -> [w663 w665]
                  tunnel: w401 -> [w662 w664]
                  frame False {
                  }
                  frame True {
                    n299 = call "Set Dev Auto.vi"("error in (no error)"=w664, "firmware revision"=w673, "dev point auto (F/F)"=w669, "VISA resource name"=w665) -> ("error out"=w672:errorcluster, "bridge error"=w670:T13, "VISA resource name out"=w671:refnum<visa-resource-name>)  [unwired: 5 in]
                    n300 = local write "bridge error"(w670) -> ()
                    n301 = call "Read Dev Auto.vi"("error in (no error)"=w672, "VISA resource name"=w671) -> ("error out"=w667:errorcluster, "dev point auto"=w668:T17, "VISA resource name out"=w666:refnum<visa-resource-name>)  [unwired: 7 in]
                    n302 = local write "dev point auto"(w668) -> ()
                  }
                }
                n303 = case shown="False" w456 {
                  tunnel: w457 -> [w651 w661]
                  tunnel: w458 -> [w650 w660]
                  tunnel: w407 -> [_ w659]
                  tunnel: w459 -> [_ w658]
                  tunnel: [w650 w653] -> w454
                  tunnel: [w651 w652] -> w455
                  frame False {
                  }
                  frame True {
                    n304 = call "Set Dev Average.vi"("error in (no error)"=w660, "firmware revision"=w659, "dev average (0)"=w658, "VISA resource name"=w661) -> ("error out"=w657:errorcluster, "bridge error"=w655:T13, "VISA resource name out"=w656:refnum<visa-resource-name>)  [unwired: 5 in]
                    n305 = local write "bridge error"(w655) -> ()
                    n306 = call "Read Dev Average.vi"("error in (no error)"=w657, "VISA resource name"=w656) -> ("error out"=w653:errorcluster, "dev average"=w654:dbl, "VISA resource name out"=w652:refnum<visa-resource-name>)  [unwired: 7 in]
                    n307 = local write "dev average"(w654) -> ()
                  }
                }
                n308 = case shown="False" w452 {
                  tunnel: w455 -> [w638 w649]
                  tunnel: w454 -> [w639 w648]
                  tunnel: [w638 w644] -> w449
                  tunnel: [w639 w642] -> w448
                  tunnel: w407 -> [_ w647]
                  tunnel: w453 -> [_ w646]
                  frame False {
                  }
                  frame True {
                    n309 = call "Set Dev Format.vi"("error in (no error)"=w648, "firmware revision"=w647, "dev format"=w646, "VISA resource name"=w649) -> ("error out"=w643:errorcluster, "bridge error"=w640:T13, "VISA resource name out"=w645:refnum<visa-resource-name>)  [unwired: 5 in]
                    n310 = local write "bridge error"(w640) -> ()
                    n311 = call "Read Dev Format.vi"("error in (no error)"=w643, "VISA resource name"=w645) -> ("error out"=w642:errorcluster, "dev format"=w641:T9, "VISA resource name out"=w644:refnum<visa-resource-name>)  [unwired: 7 in]
                    n312 = local write "dev format"(w641) -> ()
                  }
                }
                n313 = case shown="False" w450 {
                  tunnel: w449 -> [w627 w637]
                  tunnel: w448 -> [w626 w636]
                  tunnel: w407 -> [_ w635]
                  tunnel: w451 -> [_ w634]
                  tunnel: [w627 w629] -> w421
                  tunnel: [w626 w628] -> w420
                  frame False {
                  }
                  frame True {
                    n314 = call "Set Dev Rolloff.vi"("error in (no error)"=w636, "firmware revision"=w635, "dev rolloff (3000)"=w634, "VISA resource name"=w637) -> ("error out"=w632:errorcluster, "bridge error"=w633:T13, "VISA resource name out"=w631:refnum<visa-resource-name>)  [unwired: 5 in]
                    n315 = local write "bridge error"(w633) -> ()
                    n316 = call "Read Dev Rolloff.vi"("error in (no error)"=w632, "VISA resource name"=w631) -> ("error out"=w628:errorcluster, "dev rollofff"=w630:T8, "VISA resource name out"=w629:refnum<visa-resource-name>)  [unwired: 7 in]
                    n317 = local write "dev rollofff"(w630) -> ()
                  }
                }
                n318 = case shown="True" w446 {
                  tunnel: w421 -> [w590 w598]
                  tunnel: w420 -> [w589 w597]
                  tunnel: w447 -> [_ w596]
                  tunnel: w407 -> [_ w595]
                  tunnel: [w589 w592] -> w444
                  tunnel: [w590 w591] -> w445
                  frame False {
                  }
                  frame True {
                    n319 = call "Set Aout Bias.vi"("error in (no error)"=w597, "firmware revision"=w595, "aout bias"=w596, "VISA resource name"=w598) -> ("error out"=w600:errorcluster, "bridge error"=w594:T13, "VISA resource name out"=w599:refnum<visa-resource-name>)  [unwired: 5 in]
                    n320 = local write "bridge error"(w594) -> ()
                    n321 = call "Read Aout Bias.vi"("error in (no error)"=w600, "VISA resource name"=w599) -> ("error out"=w592:errorcluster, "aout bias"=w593:cluster{"ABiasC":dbl, "ABiasL":dbl}, "VISA resource name out"=w591:refnum<visa-resource-name>)  [unwired: 7 in]
                    n322 = local write "aout bias"(w593) -> ()
                  }
                }
                n323 = case shown="True" w442 {
                  tunnel: w445 -> [w581 w587]
                  tunnel: w444 -> [w580 w586]
                  tunnel: [w581 w583] -> w441
                  tunnel: [w580 w582] -> w440
                  tunnel: w407 -> [_ w585]
                  tunnel: w443 -> [_ w584]
                  frame False {
                  }
                  frame True {
                    n324 = call "Set Aout Bounds.vi"("error in (no error)"=w586, "firmware revision"=w585, "aout bounds"=w584, "VISA resource name"=w587) -> ("error out"=w582:errorcluster, "bridge error"=w588:T13, "VISA resource name out"=w583:refnum<visa-resource-name>)  [unwired: 4 in]
                    n325 = local write "bridge error"(w588) -> ()
                  }
                }
                n326 = case shown="True" w438 {
                  tunnel: w441 -> [w572 w578]
                  tunnel: w440 -> [w571 w577]
                  tunnel: [w572 w574] -> w436
                  tunnel: [w571 w573] -> w437
                  tunnel: w407 -> [_ w576]
                  tunnel: w439 -> [_ w575]
                  frame False {
                  }
                  frame True {
                    n327 = call "Set Aout Cfactor.vi"("error in (no error)"=w577, "firmware revision"=w576, "aout cfactor"=w575, "VISA resource name"=w578) -> ("error out"=w573:errorcluster, "bridge error"=w579:T13, "VISA resource name out"=w574:refnum<visa-resource-name>)  [unwired: 5 in]
                    n328 = local write "bridge error"(w579) -> ()
                  }
                }
                n329 = case shown="True" w434 {
                  tunnel: w436 -> [w563 w570]
                  tunnel: w437 -> [w562 w569]
                  tunnel: [w562 w564] -> w432
                  tunnel: [w563 w565] -> w433
                  tunnel: w407 -> [_ w567]
                  tunnel: w435 -> [_ w566]
                  frame False {
                  }
                  frame True {
                    n330 = call "Set Aout Limit.vi"("error in (no error)"=w569, "firmware revision"=w567, "aout limit"=w566, "VISA resource name"=w570) -> ("error out"=w564:errorcluster, "bridge error"=w568:T13, "VISA resource name out"=w565:refnum<visa-resource-name>)  [unwired: 5 in]
                    n331 = local write "bridge error"(w568) -> ()
                  }
                }
                n332 = case shown="True" w430 {
                  tunnel: w433 -> [w551 w559]
                  tunnel: w432 -> [w550 w558]
                  tunnel: [w551 w555] -> w429
                  tunnel: [w550 w554] -> w428
                  tunnel: w407 -> [_ w553]
                  tunnel: w431 -> [_ w552]
                  frame False {
                  }
                  frame True {
                    n333 = call "Set Aout Limit Error.vi"("error in (no error)"=w558, "firmware revision"=w553, "aout limit error"=w552, "VISA resource name"=w559) -> ("error out"=w561:errorcluster, "bridge error"=w557:T13, "VISA resource name out"=w560:refnum<visa-resource-name>)  [unwired: 5 in]
                    n334 = local write "bridge error"(w557) -> ()
                    n335 = call "Read Aout Limit Error.vi"("error in (no error)"=w561, "VISA resource name"=w560) -> ("error out"=w554:errorcluster, "aout limit error"=w556:cluster{"ALimErrC":bool, "ALimErrL":bool}, "VISA resource name out"=w555:refnum<visa-resource-name>)  [unwired: 7 in]
                    n336 = local write "aout limit error"(w556) -> ()
                  }
                }
                n337 = case shown="True" w426 {
                  tunnel: w429 -> [w542 w549]
                  tunnel: w428 -> [w541 w548]
                  tunnel: [w542 w544] -> w425
                  tunnel: [w541 w543] -> w424
                  tunnel: w407 -> [_ w547]
                  tunnel: w427 -> [_ w546]
                  frame False {
                  }
                  frame True {
                    n338 = call "Set Aout Span.vi"("error in (no error)"=w548, "firmware revision"=w547, "aout span"=w546, "VISA resource name"=w549) -> ("error out"=w543:errorcluster, "bridge error"=w545:T13, "VISA resource name out"=w544:refnum<visa-resource-name>)  [unwired: 5 in]
                    n339 = local write "bridge error"(w545) -> ()
                  }
                }
                n340 = case shown="True" w422 {
                  tunnel: w425 -> [w530 w538]
                  tunnel: w424 -> [w529 w537]
                  tunnel: [w530 w536] -> w418
                  tunnel: [w529 w535] -> w417
                  tunnel: w407 -> [_ w534]
                  tunnel: w423 -> [_ w533]
                  frame False {
                  }
                  frame True {
                    n341 = call "Set Aout Source.vi"("error in (no error)"=w537, "firmware revision"=w534, "aout source"=w533, "VISA resource name"=w538) -> ("error out"=w539:errorcluster, "bridge error"=w532:T13, "VISA resource name out"=w540:refnum<visa-resource-name>)  [unwired: 5 in]
                    n342 = local write "bridge error"(w532) -> ()
                    n343 = call "Read Aout Source.vi"("error in (no error)"=w539, "VISA resource name"=w540) -> ("error out"=w535:errorcluster, "aout source"=w531:cluster{"ASourceC":u16, "ASourceL":u16}, "VISA resource name out"=w536:refnum<visa-resource-name>)  [unwired: 7 in]
                    n344 = local write "aout source"(w531) -> ()
                  }
                }
                n345 = case shown="True" w419 {
                  tunnel: w418 -> [w601 w620]
                  tunnel: w417 -> [w602 w619]
                  tunnel: [w602 w617] -> w416
                  tunnel: [w601 w618] -> w415
                  frame False {
                  }
                  frame True {
                    n346 = call "Read Dev Parameters.vi"("error in (no error)"=w619, "VISA resource name"=w620) -> ("error out"=w606:errorcluster, "dev parameters"=w621:T18, "VISA resource name out"=w604:refnum<visa-resource-name>)  [unwired: 7 in]
                    n347 = call "Read Aout Limit.vi"("error in (no error)"=w606, "VISA resource name"=w604) -> ("error out"=w605:errorcluster, "aout limit"=w603:T20, "VISA resource name out"=w607:refnum<visa-resource-name>)  [unwired: 7 in]
                    n348 = call "Read Analog Parameters.vi"("error in (no error)"=w605, "VISA resource name"=w607) -> ("error out"=w617:errorcluster, "analog parameters"=w616:T37, "VISA resource name out"=w618:refnum<visa-resource-name>)  [unwired: 7 in]
                    n349 = Unbundle By Name(w616) -> ("aout bounds"=w611:T19, "aout cfactor"=w615:cluster{"CFactorC":dbl, "CFactorL":dbl}, "aout span"=w614:cluster{"ASpanC":dbl, "ASpanL":dbl}, "aout point"=w610:cluster{"APointC":dbl, "APointL":dbl})
                    n350 = Unbundle By Name(w621) -> ("dev point"=w612:T12, "dev bounds"=w613:T11, "dev position"=w622:T10, "dev span"=w623:cluster{"dev span cap":dbl, "dev span loss":dbl}, "dev margin"=w624:dbl)
                    n351 = local write "aout limit"(w603) -> ()
                    n352 = local write "aout bounds"(w611) -> ()
                    n353 = local write "aout cfactor"(w615) -> ()
                    n354 = local write "aout point"(w610) -> ()
                    n355 = local write "aout span"(w614) -> ()
                    n356 = local write "dev bounds"(w613) -> ()
                    n357 = local write "dev position"(w622) -> ()
                    n358 = local write "dev margin"(w624) -> ()
                    n359 = local write "dev point"(w612) -> ()
                    n360 = local write "dev span"(w623) -> ()
                    n361 = call "deviation region.vi"("dev margin"=w624, "dev bounds"=w613, "dev point"=w612) -> ("deviation region"=w625:cluster{cluster{dbl, dbl}[]}[])  [unwired: 8 in]
                    n362 = local write "deviation region"(w625) -> ()
                    n363 = call "Analog Out Region.vi"("aout limit"=w603, "aout point"=w610, "aout bounds"=w611, "dev point"=w612, "dev bounds"=w613) -> ("Loss Analog Output"=w608:cluster{cluster{dbl, dbl}[]}[], "Capacitance Analog Output"=w609:cluster{cluster{dbl, dbl}[]}[])  [unwired: 5 in]
                    n364 = local write "Capacitance Analog Output"(w609) -> ()
                    n365 = local write "Loss Analog Output"(w608) -> ()
                  }
                }
              }
              frame #2 {
                n366 = local read "bridge error"() -> (w833:T13)
                n367 = local read "measurement results"() -> (w832:T14)
                n368 = Unbundle By Name(w832) -> ("Capacitance"=→"Capacitance":dbl, "Loss"=→"Loss":dbl, "Frequency"=→"Measurement Frequency":dbl, "Voltage"=→"Applied Voltage":dbl, "GreaterThan"=w824:bool)
                n369 = local write "Measure"(FALSE ("Measure")) -> ()
                n370 = Unbundle By Name(w833) -> ("error message"=→"Error Message":string, "error code"=w827:i32)
                n371 = property on="greater than" class="Str"("Visible"=w824) -> ()  [unwired: 2 in, 2 out]
                n372 = Greater Than 0?(x=w827) -> (x > 0?=w826:bool)
                n373 = property on="Error Message" class="Str"("Visible"=w826) -> ()  [unwired: 2 in, 2 out]
              }
            }
          }
        }
        n374 = case shown="True" "Continuous" {
          tunnel: [w217 w223] -> w161
          tunnel: [w218 w222] -> w160
          tunnel: w159 -> [_ w221]
          tunnel: w89 -> [w218 w220]
          tunnel: w88 -> [w217 w219]
          frame False {
          }
          frame True {
            n375 = flat-sequence {
              tunnel: w221 -> [w248]
              tunnel: [w240] -> w223
              tunnel: [w241] -> w222
              tunnel: w220 -> [w230]
              tunnel: w219 -> [w229]
              frame #0 {
                w225 = u8 1 ("Disabled")
                n376 = property on="Measure" class="Bool (strict)"("Disabled"=w225) -> ()  [unwired: 2 in, 2 out]
                n377 = property on="Bridge Frequency" class="DigNum (strict)"("Disabled"=w225) -> ()  [unwired: 2 in, 2 out]
                n378 = property on="Average\nExponent" class="DigNum (strict)"("Disabled"=w225) -> ()  [unwired: 2 in, 2 out]
                n379 = property on="Maximum Applied Voltage" class="DigNum (strict)"("Disabled"=w225) -> ()  [unwired: 2 in, 2 out]
                n380 = property on="units" class="Ring (strict)"("Disabled"=w225) -> ()  [unwired: 2 in, 2 out]
                n381 = property on="deviation mode" class="Bool (strict)"("Disabled"=w225) -> ()  [unwired: 2 in, 2 out]
                n382 = property on="dev point" class="Clust (strict)"("Disabled"=w225) -> ()  [unwired: 2 in, 2 out]
                n383 = property on="dev span" class="Clust (strict)"("Disabled"=w225) -> ()  [unwired: 2 in, 2 out]
                n384 = property on="dev margin" class="DigNum (strict)"("Disabled"=w225) -> ()  [unwired: 2 in, 2 out]
                n385 = property on="dev bounds" class="Clust (strict)"("Disabled"=w225) -> ()  [unwired: 2 in, 2 out]
                n386 = property on="dev position" class="Clust (strict)"("Disabled"=w225) -> ()  [unwired: 2 in, 2 out]
                n387 = property on="dev fetch" class="Bool"("Disabled"=w225) -> ()  [unwired: 2 in, 2 out]
                n388 = property on="Bridge Status" class="Str"("Visible"=TRUE) -> ()  [unwired: 2 in, 2 out]
                n389 = property on="Continuous" class="Bool (strict)"("Disabled"=u8 0) -> ()  [unwired: 2 in, 2 out]
                n390 = local write "Bridge Status"("Continuous measurement" ("Bridge Status")) -> ()
                n391 = property on="dev point auto" class="Clust (strict)"("Disabled"=w225) -> ()  [unwired: 2 in, 2 out]
                n392 = property on="dev average" class="DigNum (strict)"("Disabled"=w225) -> ()  [unwired: 2 in, 2 out]
                n393 = property on="dev format" class="Clust (strict)"("Disabled"=w225) -> ()  [unwired: 2 in, 2 out]
                n394 = property on="dev rollofff" class="Clust (strict)"("Disabled"=w225) -> ()  [unwired: 2 in, 2 out]
                n395 = property on="aout bias" class="Clust (strict)"("Disabled"=w225) -> ()  [unwired: 2 in, 2 out]
                n396 = property on="aout bounds" class="Clust (strict)"("Disabled"=w225) -> ()  [unwired: 2 in, 2 out]
                n397 = property on="aout cfactor" class="Clust (strict)"("Disabled"=w225) -> ()  [unwired: 2 in, 2 out]
                n398 = property on="aout limit" class="Clust (strict)"("Disabled"=w225) -> ()  [unwired: 2 in, 2 out]
                n399 = property on="aout limit error" class="Clust (strict)"("Disabled"=w225) -> ()  [unwired: 2 in, 2 out]
                n400 = property on="aout span" class="Clust (strict)"("Disabled"=w225) -> ()  [unwired: 2 in, 2 out]
                n401 = property on="aout source" class="Clust (strict)"("Disabled"=w225) -> ()  [unwired: 2 in, 2 out]
              }
              frame #1 {
                w247 = u16 0 items=["none", "error check", "multiline read", "infinite"] ("delay")
                # "There may be an extra set of\nmeasurement results, especially\nat lower average exponent \nsettings.  Read and discard."
                n402 = local read "Average\nExponent"() -> (w235:i32)
                n403 = local read "cap graph data"() -> (w231:dbl[])
                n404 = local read "measurement buffer"() -> (w228:string[])
                n405 = local read "time graph data"() -> (w233:timestamp[])
                n406 = local read "loss graph data"() -> (w232:dbl[])
                n407 = local read "units"() -> (w234:i32)
                n408 = call "Set Continuous.vi"("error in (no error)"=w229, "continuous mode (F)"=TRUE, "VISA resource name"=w230) -> ("error out"=w253:errorcluster, "VISA resource name out"=w252:refnum<visa-resource-name>)  [unwired: 7 in]
                n409 = while {
                  tunnel: w253 -> [w277]
                  tunnel: w252 -> [w278]
                  tunnel: [w282] -> w251
                  tunnel: [w274] -> w250
                  tunnel: w248 -> [w281]
                  tunnel: [w267] -> w239
                  tunnel: [w266] -> w238
                  tunnel: [w265] -> w237
                  tunnel: [w264] -> w236
                  tunnel: w235 -> [w263]
                  tunnel: w234 -> [w262]
                  border: w231 -> [_]
                  border: w233 -> [_]
                  border: w232 -> [_]
                  border: w228 -> [_]
                  stop <- w280 stop-if-true
                  # "Process message only if\ncontinuous measurement\nhas not been cancelled\n(avoid VISA timeout)"
                  # "Wait for message in case\nof long average time"
                  n410 = while {
                    tunnel: w278 -> [w333]
                    tunnel: w277 -> [w332]
                    tunnel: [w331] -> w275
                    tunnel: [w330] -> w276
                    tunnel: [w322] -> w271
                    stop <- w327 stop-if-true
                    w326 = u16 0 items=["none", "error check", "multiline read", "infinite"] ("delay")
                    n411 = local read "Continuous"() -> (w323:bool)
                    n412 = call "Message Available.vi"("error in (no error)"=w332, "delay"=w326, "VISA resource name"=w333) -> ("error out"=w331:errorcluster, "message available"=w328:bool, "VISA resource name out"=w330:refnum<visa-resource-name>)  [unwired: 6 in]
                    n413 = local read "stop"() -> (w324:bool)
                    n414 = Not(x=w323) -> (.not. x?=w329:bool)
                    n415 = Not(x=w324) -> (.not. x?=w325:bool)
                    n416 = Compound Arithmetic op=OR(w328, w329, w324) -> (w327:bool)
                    n417 = Compound Arithmetic op=AND(w323, w325) -> (w322:bool)
                  }
                  n418 = feedback #23() -> (w269:timestamp[])
                  n419 = feedback #24() -> (w270:dbl[])
                  n420 = feedback #25() -> (w279:dbl[])
                  n421 = feedback #26() -> (w268:string[])
                  n422 = case shown="True" w271 {
                    tunnel: [w288 w321] -> w282
                    tunnel: [w287 w320] -> w274
                    tunnel: w281 -> [_ w293]
                    tunnel: w279 -> [w283 w317]
                    tunnel: [w283 w316] -> w265
                    tunnel: w269 -> [w285 w301]
                    tunnel: [w285 w302] -> w267
                    tunnel: w276 -> [w288 w314]
                    tunnel: w275 -> [w287 w315]
                    tunnel: [w286 w300] -> w266
                    tunnel: w270 -> [w286 w299]
                    tunnel: w263 -> [_ w296]
                    tunnel: w262 -> [_ w294]
                    tunnel: [w284 w290] -> w264
                    tunnel: w268 -> [w284 w289]
                    frame False {
                    }
                    frame True {
                      w310 = u16 0 items=["Single Line", "Multi-Line"] ("Multiline")
                      n423 = Get Date/Time In Seconds() -> (seconds since 1Jan1904=w292:timestamp)
                      n424 = call "Bridge Read.vi"("error in (no error)"=w315, "multiline"=w310, "VISA resource name"=w314) -> ("error out"=w312:errorcluster, "read buffer"=w311:string, "VISA resource name out"=w313:refnum<visa-resource-name>)  [unwired: 6 in]
                      n425 = call "Parse Results.vi"("measurement line"=w311) -> ("measurement results"=w295:T38)  [unwired: 9 in]
                      n426 = Unbundle By Name(w295) -> ("frequency"=w306:dbl, "capacitance"=w307:dbl, "greater than"=w304:bool, "loss"=w303:dbl, "voltage"=w305:dbl)
                      n427 = call "Error Query.vi"("error in (no error)"=w312, "firmware revision"=w293, "measurement line"=w311, "VISA resource name"=w313) -> ("error out"=w320:errorcluster, "bridge error"=w319:T13, "VISA resource name out"=w321:refnum<visa-resource-name>)  [unwired: 5 in]
                      n428 = Unbundle By Name(w319) -> ("error message"=w318:string, "error code"=w308:i32)
                      n429 = call "Log Line.vi"("average exponent"=w296, "current time"=w292, "firmware revision"=w293, "units"=w294, "measurement results"=w295) -> ("log line"=w291:string)  [unwired: 6 in]
                      n430 = Insert Into Array(array=w289, new element=w291) -> (w290:string[])  [unwired: 1 in]
                      n431 = Insert Into Array(array=w317, new element=w307) -> (w316:dbl[])  [unwired: 1 in]
                      n432 = Insert Into Array(array=w299, new element=w303) -> (w300:dbl[])  [unwired: 1 in]
                      n433 = Insert Into Array(array=w301, new element=w292) -> (w302:timestamp[])  [unwired: 1 in]
                      n434 = local write "Error Message"(w318) -> ()
                      n435 = Greater Than 0?(x=w308) -> (x > 0?=w309:bool)
                      n436 = property on="Error Message" class="Str"("Visible"=w309) -> ()  [unwired: 2 in, 2 out]
                      n437 = Bundle("time graph data"=w302, "cap graph data"=w316) -> (w298:T35)  [unwired: 1 in]
                      n438 = Bundle("time graph data"=w302, "loss graph data"=w300) -> (w297:T36)  [unwired: 1 in]
                      n439 = local write "Measurement Frequency"(w306) -> ()
                      n440 = local write "Capacitance"(w307) -> ()
                      n441 = local write "Applied Voltage"(w305) -> ()
                      n442 = local write "Loss"(w303) -> ()
                      n443 = property on="greater than" class="Str"("Visible"=w304) -> ()  [unwired: 2 in, 2 out]
                      n444 = local write "Capacitance Graph"(w298) -> ()
                      n445 = local write "Loss Graph"(w297) -> ()
                    }
                  }
                  n446 = feedback-in #23(w267) -> ()
                  n447 = feedback-in #24(w266) -> ()
                  n448 = feedback-in #25(w265) -> ()
                  n449 = feedback-in #26(w264) -> ()
                  n450 = Unbundle By Name(w274) -> ("status"=w273:bool)
                  n451 = Not(x=w271) -> (.not. x?=w272:bool)
                  n452 = Compound Arithmetic op=OR(w273, w272) -> (w280:bool)
                }
                n453 = local write "cap graph data"(w237) -> ()
                n454 = local write "measurement buffer"(w236) -> ()
                n455 = local write "time graph data"(w239) -> ()
                n456 = local write "loss graph data"(w238) -> ()
                n457 = call "Set Continuous.vi"("error in (no error)"=w250, "continuous mode (F)"=FALSE, "VISA resource name"=w251) -> ("error out"=w242:errorcluster, "VISA resource name out"=w243:refnum<visa-resource-name>)  [unwired: 7 in]
                n458 = call "Message Available.vi"("error in (no error)"=w242, "delay"=w247, "VISA resource name"=w243) -> ("error out"=w245:errorcluster, "message available"=w244:bool, "VISA resource name out"=w246:refnum<visa-resource-name>)  [unwired: 6 in]
                n459 = case shown="True" w244 {
                  tunnel: w246 -> [w256 w260]
                  tunnel: w245 -> [w255 w259]
                  tunnel: [w256 w258] -> w241
                  tunnel: [w255 w257] -> w240
                  frame False {
                  }
                  frame True {
                    w261 = u16 1 items=["Single Line", "Multi-Line"] ("Multiline")
                    n460 = call "Bridge Read.vi"("error in (no error)"=w259, "multiline"=w261, "VISA resource name"=w260) -> ("error out"=w257:errorcluster, "VISA resource name out"=w258:refnum<visa-resource-name>)  [unwired: 6 in, 1 out]
                  }
                }
              }
            }
          }
        }
        n461 = Unbundle By Name(w161) -> ("code"=w199:i32)
        n462 = Equal?(x=w199, y=-1074000000 ("Code")) -> (x = y?=w197:bool)
        n463 = case shown="False" w197 {
          tunnel: w161 -> [w835 w837]
          tunnel: [w835 w836] -> w196
          frame False {
          }
          frame True {
            n464 = call <vilib>:"Clear Errors.vi"("error in (no error)"=w837) -> ("error out"=w836:errorcluster)  [unwired: 5 in, 1 out]
          }
        }
        n465 = call <vilib>:"Simple Error Handler.vi"("error in (no error)"=w196) -> ("error?"=w207:bool, "error out"=w204:errorcluster)  [unwired: 4 in, 3 out]
        n466 = Or(x=w207, y="stop") -> (x .or. y?=w205:bool)
        n467 = property on="Bridge Status" class="Str"("Visible"=FALSE) -> ()  [unwired: 2 in, 2 out]
        n468 = property on="Measure" class="Bool (strict)"("Disabled"=w102) -> ()  [unwired: 2 in, 2 out]
        n469 = property on="Bridge Frequency" class="DigNum (strict)"("Disabled"=w102) -> ()  [unwired: 2 in, 2 out]
        n470 = property on="Average\nExponent" class="DigNum (strict)"("Disabled"=w102) -> ()  [unwired: 2 in, 2 out]
        n471 = property on="Maximum Applied Voltage" class="DigNum (strict)"("Disabled"=w102) -> ()  [unwired: 2 in, 2 out]
        n472 = property on="units" class="Ring (strict)"("Disabled"=w102) -> ()  [unwired: 2 in, 2 out]
        n473 = property on="deviation mode" class="Bool (strict)"("Disabled"=w102) -> ()  [unwired: 2 in, 2 out]
        n474 = property on="dev point" class="Clust (strict)"("Disabled"=w102) -> ()  [unwired: 2 in, 2 out]
        n475 = property on="dev span" class="Clust (strict)"("Disabled"=w102) -> ()  [unwired: 2 in, 2 out]
        n476 = property on="dev margin" class="DigNum (strict)"("Disabled"=w102) -> ()  [unwired: 2 in, 2 out]
        n477 = property on="dev bounds" class="Clust (strict)"("Disabled"=w102) -> ()  [unwired: 2 in, 2 out]
        n478 = property on="dev position" class="Clust (strict)"("Disabled"=w102) -> ()  [unwired: 2 in, 2 out]
        n479 = property on="dev fetch" class="Bool"("Disabled"=w102) -> ()  [unwired: 2 in, 2 out]
        n480 = property on="dev point auto" class="Clust (strict)"("Disabled"=w102) -> ()  [unwired: 2 in, 2 out]
        n481 = property on="dev average" class="DigNum (strict)"("Disabled"=w102) -> ()  [unwired: 2 in, 2 out]
        n482 = property on="dev format" class="Clust (strict)"("Disabled"=w102) -> ()  [unwired: 2 in, 2 out]
        n483 = property on="dev rollofff" class="Clust (strict)"("Disabled"=w102) -> ()  [unwired: 2 in, 2 out]
        n484 = property on="Continuous" class="Bool (strict)"("Disabled"=w102) -> ()  [unwired: 2 in, 2 out]
        n485 = property on="aout bias" class="Clust (strict)"("Disabled"=w102) -> ()  [unwired: 2 in, 2 out]
        n486 = property on="aout bounds" class="Clust (strict)"("Disabled"=w102) -> ()  [unwired: 2 in, 2 out]
        n487 = property on="aout cfactor" class="Clust (strict)"("Disabled"=w102) -> ()  [unwired: 2 in, 2 out]
        n488 = property on="aout limit" class="Clust (strict)"("Disabled"=w102) -> ()  [unwired: 2 in, 2 out]
        n489 = property on="aout limit error" class="Clust (strict)"("Disabled"=w102) -> ()  [unwired: 2 in, 2 out]
        n490 = property on="aout span" class="Clust (strict)"("Disabled"=w102) -> ()  [unwired: 2 in, 2 out]
        n491 = property on="aout source" class="Clust (strict)"("Disabled"=w102) -> ()  [unwired: 2 in, 2 out]
      }
    }
  }
  n492 = while {
    stop <- w838 stop-if-true
    n493 = local read "deviation mode"() -> (w843:bool)
    n494 = local read "Measure"() -> (w839:bool)
    n495 = local read "stop"() -> (w838:bool)
    n496 = Not(x=w843) -> (.not. x?=w842:bool)
    n497 = Or(x=w842, y=w838) -> (x .or. y?=w841:bool)
    n498 = Or(x=w839, y=w838) -> (x .or. y?=w840:bool)
    n499 = local write "cancel measure"(w840) -> ()
    n500 = local write "cancel dev init"(w841) -> ()
  }
  n501 = call "Close.vi"("error in (no error)"=w60, "VISA resource name"=w59) -> ()  [unwired: 9 in, 1 out]
  "pF" <- "pF" ("pF")
  "Hz" <- w43
  "V" <- w42
  "Hz 2" <- w43
  "V 2" <- w42
